vi "OC2 init.vi"(2 "error in (no error)":errorcluster, 3 "VISA resource name":refnum<visa-resource-name>) -> (0 "error out":errorcluster, 1 "duplicate VISA resource name":refnum<visa-resource-name>)   [LabVIEW 2009]
uses:
  <vilib>/Instr/_visa.llb/VISA Configure Serial Port (Instr).vi
panel:
  in  "baud rate":u32
  # "Initialise"
  # "V1.02"
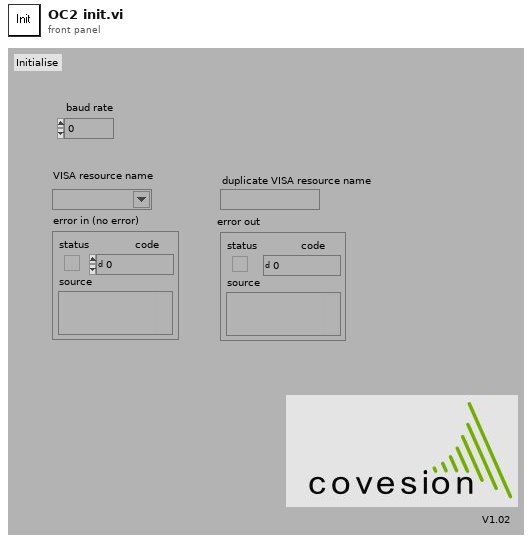
[diagram p1: front panel]
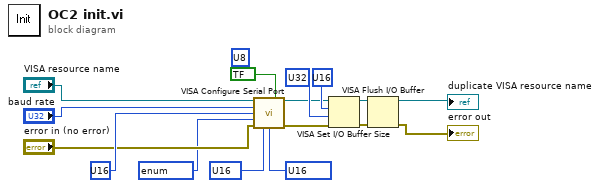
[diagram p0: block diagram]
diagram:
  (unwired) u8 ? ("termination char\n(0xA = '\\n' = LF)")
  w9 = u16 ? items=["1.0", "1.5", "2.0"] ("stop bits (10: 1 bit)")
  w11 = u16 ? items=["None", "XON/XOFF", "RTS/CTS", "XON/XOFF & RTS/CTS", "DTR/DSR", "XON/XOFF & DTR/DSR"] ("flow control (0:none)")
  n1 = call-poly "VISA Configure Serial Port"("VISA resource name"="VISA resource name", "Enable Termination\nChar (T)"=bool ? ("Enable Termination\nChar (T)"), "baud rate (9600)"="baud rate", "data bits (8)"=u16 ? ("data bits"), "parity (0:none)"=enum16{"None", "Odd", "Even", "Mark", "Space"} ?, "error in (no error)"="error in (no error)", "stop bits (10: 1 bit)"=w9, "flow control (0:none)"=w11) -> ("VISA resource name out"=w3:refnum<visa-resource-name>, "error out"=w4:errorcluster)  [unwired: 6 in]
  n2 = VISA Set I/O Buffer Size(VISA resource name=w3, mask (16)=u16 ?, size (4096)=u32 ?, error in (no error)=w4) -> (VISA resource name out=w8:refnum<visa-resource-name>, error out=w7:errorcluster)
  n3 = VISA Flush I/O Buffer(VISA resource name=w8, error in (no error)=w7) -> (VISA resource name out=→"duplicate VISA resource name":refnum<visa-resource-name>, error out=→"error out":errorcluster)  [unwired: 1 in]
